vi "RSZVB Define Port Pair.vi"(5 "Port 2 (2)":i32=2, 6 "Port 1 (1)":i32=1, 7 "Port Pair (1)":i32=1, 8 "error in (no error)":errorcluster {"code" format="%.0x"}, 9 "Function Type (Deembedding)":i32(ring) items=["Deembedding", "Embedding"], 10 "Channel (1)":i32=1, 11 "VISA session":refnum<visa-resource-name>) -> (0 "error out":errorcluster {"code" format="%.0x"}, 3 "dup VISA session":refnum<visa-resource-name>)   [LabVIEW 2011]
doc: "Defines a list of port pairs for port pair deembedding/embedding. The command can be used repeatedly to extend or overwrite the list.\n\nRemote-control command(s):\nCALCulate<Ch>:TRANsform:VNETworks:PPAir:DEEMbedding<List_idx>:DEFine\nCALCulate<Ch>:TRANsform:VNETworks:PPAir:EMBedding<List_idx>:DEFine"
uses:
  _utility/RSZVB Global Data.vi
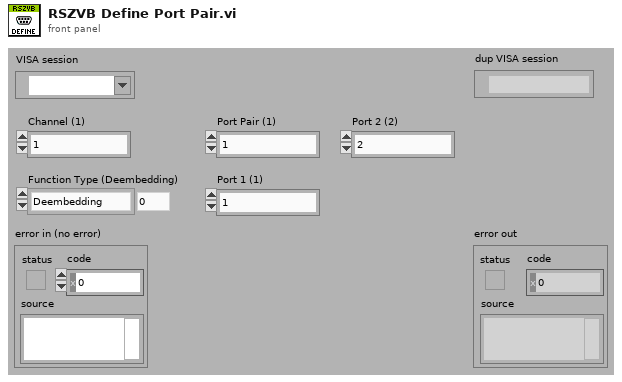
[diagram p1: front panel]
types:
  T1 = cluster{"Error Checking (T: On)":bool, "Installed Options":string[], "Data Valid?":bool, "Ports":i32, "Model":string[], "Option Checking (T: On)":bool}[]
  T2 = cluster{"Error Checking (T: On)":bool, "Installed Options":string[], "Data Valid?":bool, "Ports":i32, "Model":string[], "Option Checking (T: On)":bool}
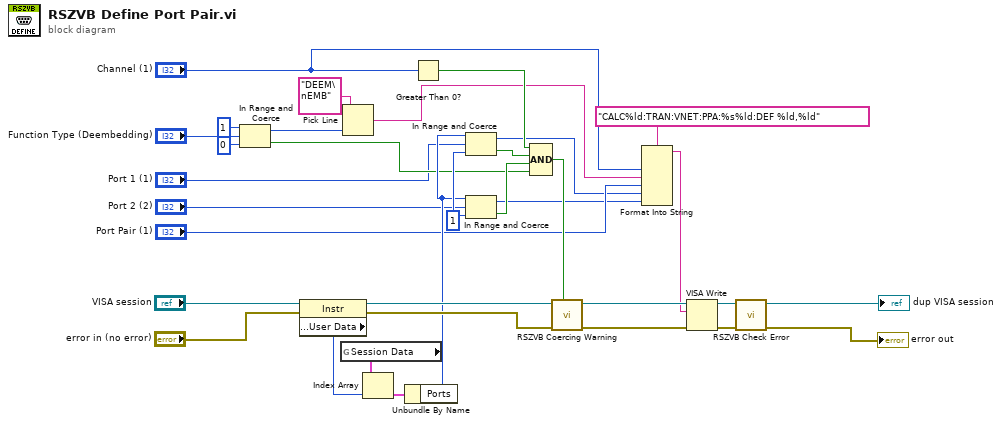
[diagram p0: block diagram]
diagram:
  w10 = 1 ("lower limit")
  n1 = In Range and Coerce(upper limit=1, x="Function Type (Deembedding)", lower limit=0) -> (coerced(x)=w12:i32, In Range?=w6:bool)
  n2 = property class="Instr"(reference="VISA session", error in="error in (no error)") -> (reference out=w34:refnum<visa-resource-name>, error out=w33:errorcluster, "General Settings:User Data"=w32:u32)
  n3 = global read "RSZVB Global Data.vi" "Session Data"() -> (w31:T1)
  n4 = Pick Line(multi-line string="DEEM\nEMB", line index=w12) -> (output string=w11:string)  [unwired: 1 in]
  n5 = Index Array(array=w31, index=w32) -> (element=w30:T2)
  n6 = Unbundle By Name(w30) -> ("Ports"=w9:i32)
  n7 = Greater Than 0?(x="Channel (1)") -> (x > 0?=w29:bool)
  n8 = In Range and Coerce(upper limit=w9, x="Port 1 (1)", lower limit=w10) -> (coerced(x)=w2:i32, In Range?=w8:bool)
  n9 = In Range and Coerce(upper limit=w9, x="Port 2 (2)", lower limit=w10) -> (coerced(x)=w1:i32, In Range?=w7:bool)
  n10 = Compound Arithmetic op=AND(w29, w8, w7, w6) -> (w28:bool)
  n11 = call "RSZVB Coercing Warning.vi"("In Range?"=w28, "error in (no error)"=w33, "VISA session"=w34) -> ("error out"=w25:errorcluster, "dup VISA session"=w24:refnum<visa-resource-name>)  [unwired: 7 in]
  n12 = Format Into String(format string="CALC%ld:TRAN:VNET:PPA:%s%ld:DEF %ld,%ld", "Channel (1)", w11, "Port Pair (1)", w2, w1) -> (resulting string=w23:string)  [unwired: 2 in, 1 out]
  n13 = VISA Write(VISA resource name=w24, write buffer=w23, error in (no error)=w25) -> (VISA resource name out=w27:refnum<visa-resource-name>, error out=w26:errorcluster)  [unwired: 1 out]
  n14 = call "RSZVB Check Error.vi"("error in (no error)"=w26, "VISA session"=w27) -> ("error out"=→"error out":errorcluster, "dup VISA session"=→"dup VISA session":refnum<visa-resource-name>)  [unwired: 8 in]
